vi "Generador_Funciones.vi"() -> ()   [LabVIEW 2016]
panel:
  out "Waveform Chart":dbl(graph)
  in  "Enum":T1(ring)
  out "Numeric Control":dbl
  in  "Stop Button":bool
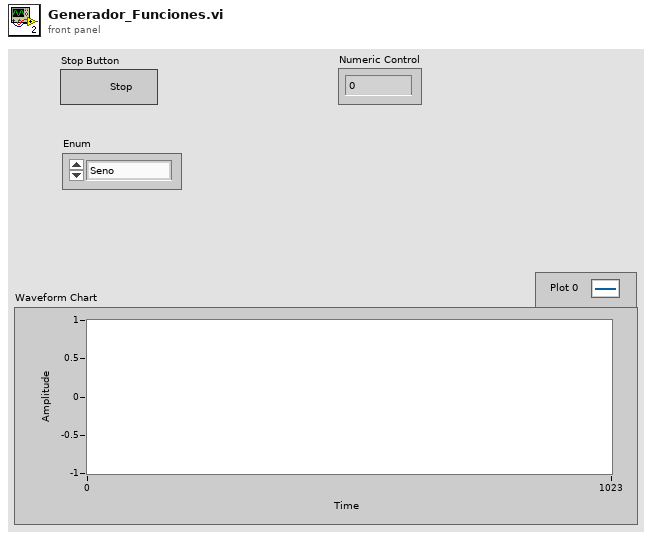
[diagram p1: front panel]
types:
  T1 = enum16{"Seno", "Triangular", "Diente de Sierra", "Pulso", "Secante", "DC", "GND"}
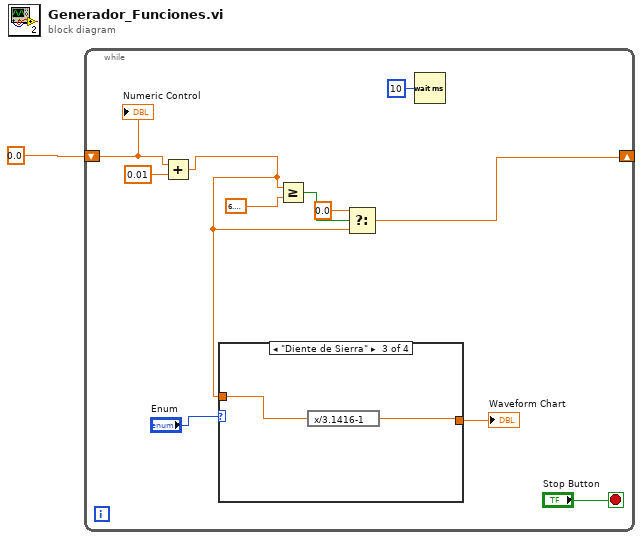
[diagram p0: block diagram]
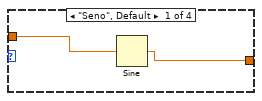
[diagram p2: hidden frame]
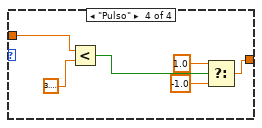
[diagram p4: hidden frame]
diagram:
  n1 = while {
    shift-right: [w5] -> _
    shift-left: 0.0 -> [w12]
    stop <- "Stop Button" stop-if-true
    n2 = Add(x=w12, y=0.01) -> (x+y=w3:dbl)
    n3 = case shown="\"Diente de Sierra\"" "Enum" {
      tunnel: w3 -> [w14 _ w16 w21]
      tunnel: [w13 _ w15 w17] -> w2
      frame "Seno", Default {
        n4 = Sine(x=w14) -> (sin(x)=w13:dbl)
      }
      frame "Triangular" {
      }
      frame "Diente de Sierra" {
        n5 = expression code="x/3.1416-1"(w16) -> (w15:dbl)
      }
      frame "Pulso" {
        n6 = Less?(x=w21, y=3.141592653589793) -> (x < y?=w22:bool)
        n7 = Select(t=1.0, s=w22, f=-1.0) -> (s? t:f=w17:dbl)
      }
    }
    "Waveform Chart" <- w2
    n8 = Greater Or Equal?(x=w3, y=6.283185307179586) -> (x >= y?=w7:bool)
    n9 = Select(t=0.0, s=w7, f=w3) -> (s? t:f=w5:dbl)
    n10 = Wait (ms)(milliseconds to wait=u32 10) -> ()  [unwired: 1 out]
    "Numeric Control" <- w12
  }
